vi "Handle.vi"(8 "Error In":errorcluster, 9 "Action":string, 10 "Values":dbl[](array[numeric]), 11 "reference in":refnum<class "BaseHandler.lvclass">) -> (0 "Error Out":errorcluster, 2 "Return(DBL)":dbl, 3 "reference out":refnum<class "BaseHandler.lvclass">)   [LabVIEW 2020, in "BaseHandler.lvclass"]
uses:
  BaseHandler.lvclass
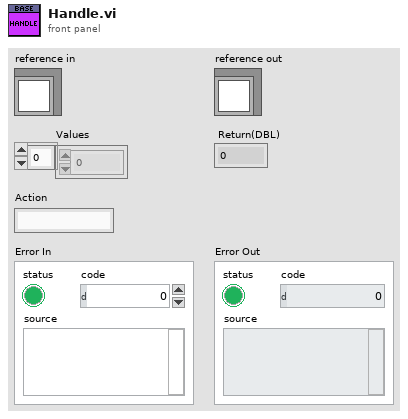
[diagram p1: front panel]
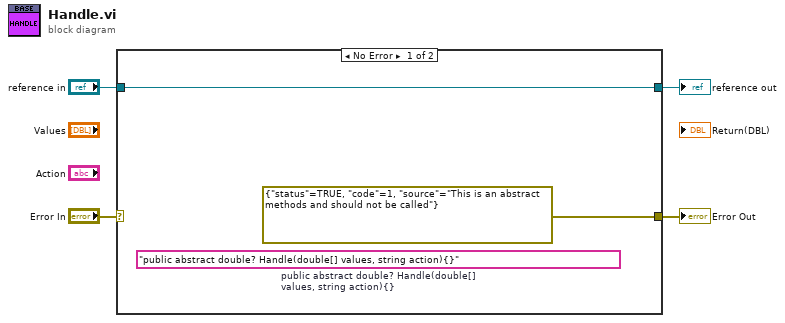
[diagram p0: block diagram]
diagram:
  n1 = case shown="No Error" "Error In" {
    selector: "Error In" -> [_ w8]
    tunnel: [errorcluster {"status"=TRUE, "code"=1, "source"="This is an abstract methods and should not be called"} ("error IO") w8] -> w3
    tunnel: [w5 w7] -> w1
    tunnel: "reference in" -> [w5 w7]
    frame No Error {
      (unwired) "public abstract double? Handle(double[] values, string action){}"  # public abstract double? Handle(double[] values, string action){}
    }
    frame Error {
    }
  }
  "Error Out" <- w3
  "reference out" <- w1
